vi "daqio_Connect_Device.vi"(4 "Buffer Settings":T1={"Max File Size (Bytes)"=100000, "Save File after no of Writes"=100, "Timeout"=10000}, 6 "daq.io API base":string="http://development.daq.io/api/v2", 7 "Device Specifier":T2, 8 "error in (no error)":errorcluster, 9 "Device Token":string, 10 "Credentials":T5, 11 "Use System Status Event?":bool=TRUE) -> (0 "error out":errorcluster, 1 "connected successfully?":bool, 3 "daq.io type out":T3={"daq.io ref"=refnum, "daq.io API Base"="http://dashboard.daq.io/api/v1", "Device Key"="", "Account ID"="", "online"=TRUE, "SSL"=FALSE})   [LabVIEW 2013, in "daqio minimal.lvlib"]
doc: "This VI connects the current device (the one the VI is executed on) to the daq.io cloud connection.\nPlease refer to a \"Device Key\". If the selected \"Device Key\" does not exist, it will be created by daq.io. If \"Device Key\" is left blank, the machine's host name will be used as a device name and appear that way online.\n\nUse the Buffer Settings to adjust the internal data buffer for intermittent connection. \n\nIf \"Use System Status Event?\" is True, then an Event Type will be generated that is call \"System Status\" and that can be used for connectivity status information."
uses:
  daqio minimal.lvlib
  _typedefs/daqio-Credentials.ctl
  _typedefs/daqio-Type.ctl
  <vilib>/httpClient/ClientHandle.ctl
  _typedefs/daqio-Device-Specifier.ctl
  _typedefs/daqio-Buffer-Parameters.ctl
  _typedefs/connection_FGV_commands.ctl
  _typedefs/daqio-reconnect-status.ctl
  _typedefs/daqio-Buffer-Commands.ctl
  <vilib>/httpClient/LabVIEWHTTPClient.lvlib
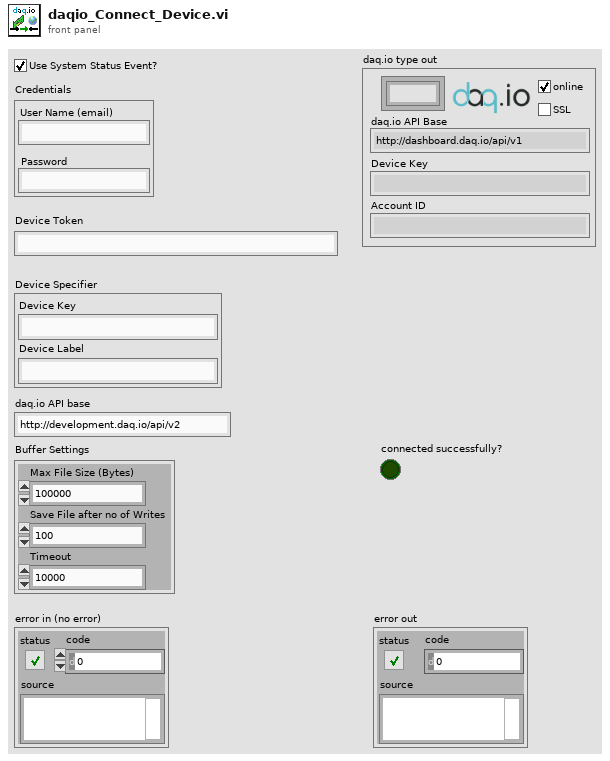
[diagram p1: front panel]
types:
  T1 = typedef "daqio minimal.lvlib/daqio-Buffer-Parameters.ctl" = cluster{"Max File Size (Bytes)":i32, "Save File after no of Writes":i32, "Timeout":i32}
  T2 = typedef "daqio minimal.lvlib/daqio-Device-Specifier.ctl" = cluster{"Device Key":string, "Device Label":string}
  T3 = typedef "daqio minimal.lvlib/daqio-Type.ctl" = cluster{"daq.io ref":T4, "daq.io API Base":string, "Device Key":string, "Account ID":string, "online":bool, "SSL":bool}
  T4 = typedef "LabVIEWHTTPClient.lvlib/ClientHandle.ctl" = refnum<k1>
  T5 = typedef "daqio minimal.lvlib/daqio-Credentials.ctl" = cluster{"User Name (email)":string, "Password":string}
  T6 = typedef "daqio minimal.lvlib/connection_FGV_commands.ctl" = enum16{"Set Conn Stat", "Save Type", "Get Type from File", "Set Type", "Set Buffer", "Get"}
  T7 = typedef "daqio minimal.lvlib/daqio-reconnect-status.ctl" = enum16{"Reconnect success", "Reconnect failed", "Connected", "Offline"}
  T8 = typedef "daqio minimal.lvlib/daqio-Buffer-Commands.ctl" = enum16{"Add to Buffer", "Post from Buffer", "Clear Buffer", "Init"}
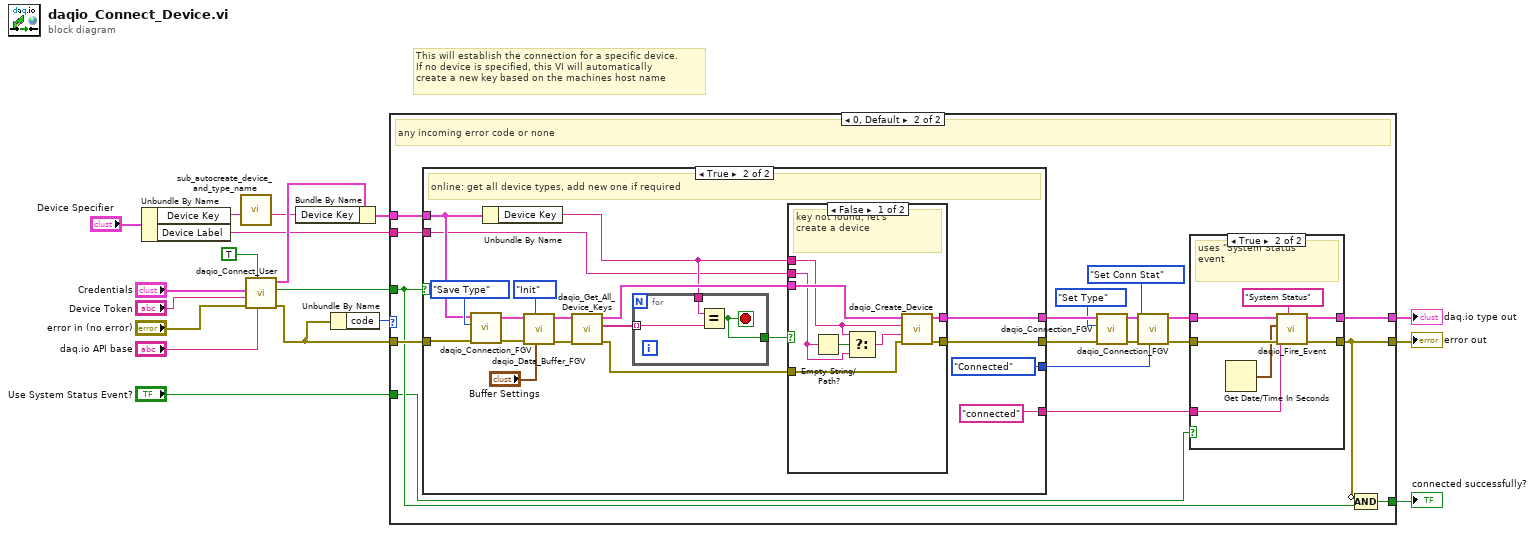
[diagram p0: block diagram]
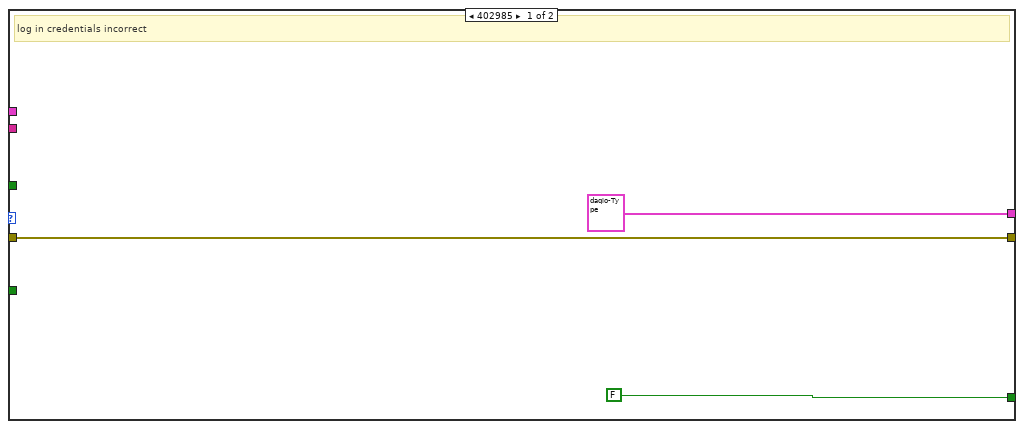
[diagram p2: hidden frame]
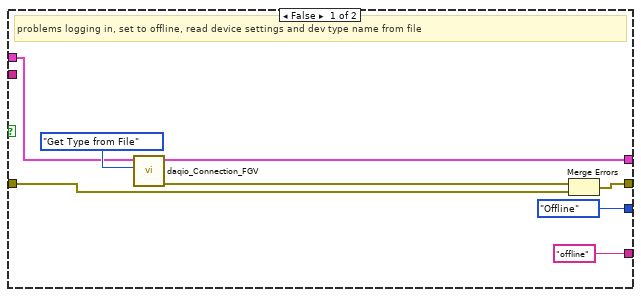
[diagram p4: hidden frame]
diagram:
  # "This will establish the connection for a specific device. \nIf no device is specified, this VI will automatically\ncreate a new key based on the machines host name"
  n1 = Unbundle By Name("Device Specifier") -> ("Device Key"=w13:string, "Device Label"=w4:string)
  n2 = call "sub_autocreate_device_and_type_name.vi"("Device_Key in"=w13) -> ("Device_Key out"=w12:string)  [unwired: 10 in]
  n3 = call "daqio_Connect_User.vi"("daq.io API base"="daq.io API base", "Use SSL"=TRUE, "error in (no error)"="error in (no error)", "Device Token"="Device Token", "Credentials"="Credentials") -> ("error out"=w5:errorcluster, "logged in?"=w11:bool, "daq.io type"=w16:T3)  [unwired: 4 in]
  n4 = Bundle By Name(cluster=w16, "Device Key"=w12) -> (w15:T3)
  n5 = Unbundle By Name(w5) -> ("code"=w6:i32)
  n6 = case shown="0, Default" w6 {
    tunnel: w5 -> [w21 w39]
    tunnel: w15 -> [_ w38]
    tunnel: w11 -> [_ w37]
    tunnel: [FALSE w36] -> w10
    tunnel: [w21 w32] -> w9
    tunnel: [T3 {"daq.io ref"=refnum, "daq.io API Base"="http://dashboard.daq.io/api/v1", "Device Key"="", "Account ID"="", "online"=FALSE, "SSL"=TRUE} ("daq.io type out") w31] -> w8
    tunnel: "Use System Status Event?" -> [_ w30]
    tunnel: w4 -> [_ w22]
    frame 402985 {
      # "log in credentials incorrect"
    }
    frame 0, Default {
      # "any incoming error code or none"
      n7 = case shown="True" w37 {
        tunnel: w38 -> [w53 w65]
        tunnel: w39 -> [w51 w64]
        tunnel: [w49 w74] -> w33
        tunnel: [w52 w73] -> w35
        tunnel: [daqio-reconnect-status."Offline" ("Connection Status in") daqio-reconnect-status."Connected" ("Connection Status in")] -> w24
        tunnel: ["offline" ("Event Value") "connected" ("Event Value")] -> w23
        tunnel: w22 -> [_ w57]
        frame False {
          # "problems logging in, set to offline, read device settings and dev type name from file"
          n8 = call "daqio_Connection_FGV.vi"("Enum"=connection_FGV_commands."Get Type from File", "daq.io type in"=w53) -> ("error out"=w50:errorcluster, "daq.io type out"=w52:T3)  [unwired: 6 in, 2 out]
          n9 = Merge Errors(w50, w51) -> (w49:errorcluster)
        }
        frame True {
          # "online: get all device types, add new one if required"
          n10 = call "daqio_Connection_FGV.vi"("error in"=w64, "Enum"=connection_FGV_commands."Save Type", "daq.io type in"=w65) -> ("error out"=w63:errorcluster, "daq.io type out"=w62:T3)  [unwired: 5 in, 2 out]
          n11 = Unbundle By Name(w65) -> ("Device Key"=w60:string)
          n12 = call "daqio_Data_Buffer_FGV.vi"("Buffer Settings"="Buffer Settings", "Buffer Command"=daqio-Buffer-Commands."Init", "error in (no error)"=w63, "daq.io type in"=w62) -> ("error out"=w72:errorcluster, "daq.io type out"=w71:T3)  [unwired: 6 in]
          n13 = call "daqio_Get_All_Device_Keys.vi"("error in"=w72, "daq.io type in"=w71) -> ("error out"=w58:errorcluster, "Existing Device Keys"=w61:string[], "daq.io type out"=w75:T3)  [unwired: 7 in]
          n14 = for {
            tunnel: w61 -> [w76] mode=indexing
            tunnel: w60 -> [w78]
            tunnel: [w77] -> w59
            stop <- w77 stop-if-true
            n15 = Equal?(x=w78, y=w76) -> (x = y?=w77:bool)
          }
          n16 = case shown="False" w59 {
            tunnel: w60 -> [w80 _]
            tunnel: w75 -> [w86 w88]
            tunnel: [w83 w87] -> w74
            tunnel: [w84 w88] -> w73
            tunnel: w58 -> [w85 w87]
            tunnel: w57 -> [w81 _]
            frame False {
              # "key not found, let's \ncreate a device"
              n17 = Empty String/Path?(string/path=w81) -> (empty?=w82:bool)
              n18 = Select(t=w80, s=w82, f=w81) -> (s? t:f=w79:string)
              n19 = call "daqio_Create_Device.vi"("error in"=w85, "Device Label"=w79, "Device Key"=w80, "daq.io type in"=w86) -> ("error out"=w83:errorcluster, "daq.io type out"=w84:T3)  [unwired: 6 in]
            }
            frame True {
              # "nothing to do"
            }
          }
        }
      }
      n20 = call "daqio_Connection_FGV.vi"("error in"=w33, "Enum"=connection_FGV_commands."Set Type", "daq.io type in"=w35) -> ("error out"=w28:errorcluster, "daq.io type out"=w29:T3)  [unwired: 5 in, 2 out]
      n21 = call "daqio_Connection_FGV.vi"("Connection Status in"=w24, "error in"=w28, "Enum"=connection_FGV_commands."Set Conn Stat", "daq.io type in"=w29) -> ("error out"=w27:errorcluster, "daq.io type out"=w26:T3)  [unwired: 4 in, 2 out]
      n22 = case shown="True" w30 {
        tunnel: w26 -> [w41 w48]
        tunnel: w27 -> [w40 w47]
        tunnel: [w40 w44] -> w32
        tunnel: [w41 w43] -> w31
        tunnel: w23 -> [_ w42]
        frame False {
        }
        frame True {
          # "uses \"System Status\"\nevent"
          n23 = Get Date/Time In Seconds() -> (seconds since 1Jan1904=w46:timestamp)
          n24 = call "daqio_Fire_Event.vi"("Event Key"="System Status", "error in (no error)"=w47, "Event Value"=w42, "Event Date and Time"=w46, "daq.io type in"=w48) -> ("error out"=w44:errorcluster, "daq.io type out"=w43:T3)  [unwired: 5 in]
        }
      }
      n25 = Compound Arithmetic op=AND(invert w32, w37) -> (w36:bool)
    }
  }
  "error out" <- w9
  "daq.io type out" <- w8
  "connected successfully?" <- w10
